vi "FakeFact.vi"() -> (0 "error out":errorcluster)   [LabVIEW 2019, in "TestCaseTest.lvlib" / "Support.lvlib"]
uses:
  Support.lvlib
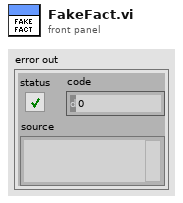
[diagram p1: front panel]
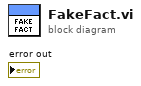
[diagram p0: block diagram]
diagram:
